vi "Manage_Database.vi"(8 "error in":errorcluster, 10 "To_Do":T1, 11 "All_Communication IN":T2 {"ConfigurationDatabase"."InactivityTime" format="%.0f seconds"; "ConfigurationDatabase"."TravelTime" format="%.0f seconds"; "ConfigurationDatabase"."DoorClose" format="%.0f seconds"; "ConfigurationDatabase"."DoorOpen" format="%.0f seconds"}) -> (0 "error out":errorcluster, 3 "All_Communication OUT":T2 {"ConfigurationDatabase"."InactivityTime" format="%.0f seconds"; "ConfigurationDatabase"."TravelTime" format="%.0f seconds"; "ConfigurationDatabase"."DoorClose" format="%.0f seconds"; "ConfigurationDatabase"."DoorOpen" format="%.0f seconds"})   [LabVIEW 2020]
doc: "Read XML Database, if there is not file load default conf"
uses:
  controls/All_Communication_Data.ctl
  controls/Configuration_Database.ctl
  Message Queue/All Message Queues.ctl
  Message Queue/Message Cluster.ctl
  controls/Event_User.ctl
  Controls/DB_To_do.ctl
  <vilib>/Utility/xml.llb/Write to XML File(string).vi
  <vilib>/Utility/xml.llb/Read From XML File(string).vi
  Message Queue/Message Queue.lvlib
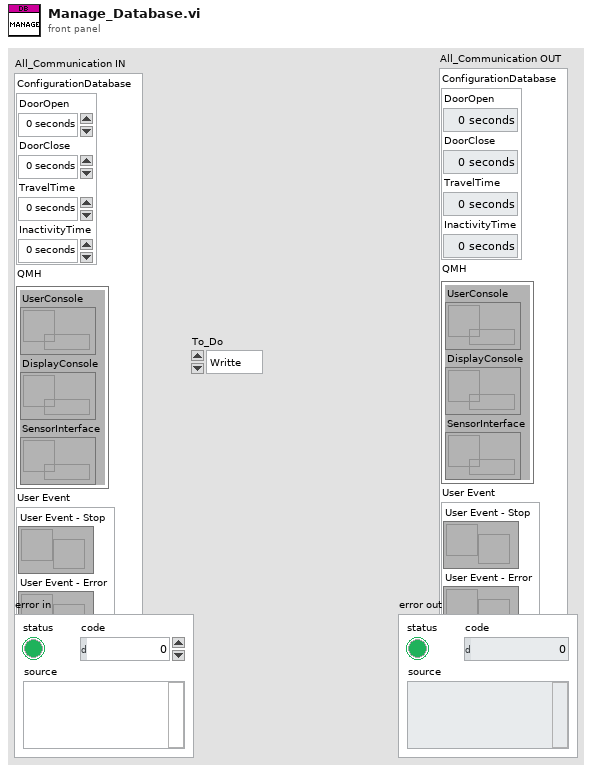
[diagram p1: front panel]
types:
  T1 = typedef "DB_To_do.ctl" = enum16{"Writte", "Read"}
  T2 = typedef "All_Communication_Data.ctl" = cluster{"ConfigurationDatabase":T3, "QMH":T4, "User Event":T5}
  T3 = typedef "Configuration_Database.ctl" = cluster{"DoorOpen":u8, "DoorClose":u8, "TravelTime":u8, "InactivityTime":u8}
  T4 = typedef "Message Queue.lvlib/All Message Queues.ctl" = cluster{"UserConsole":refnum<queue>, "DisplayConsole":refnum<queue>, "SensorInterface":refnum<queue>}
  T5 = typedef "Event_User.ctl" = cluster{"User Event - Stop":refnum<user-event>, "User Event - Error":refnum<user-event>}
  T6 = enum16{"open", "replace", "create", "open or create", "replace or create", "replace or create with confirmation"}
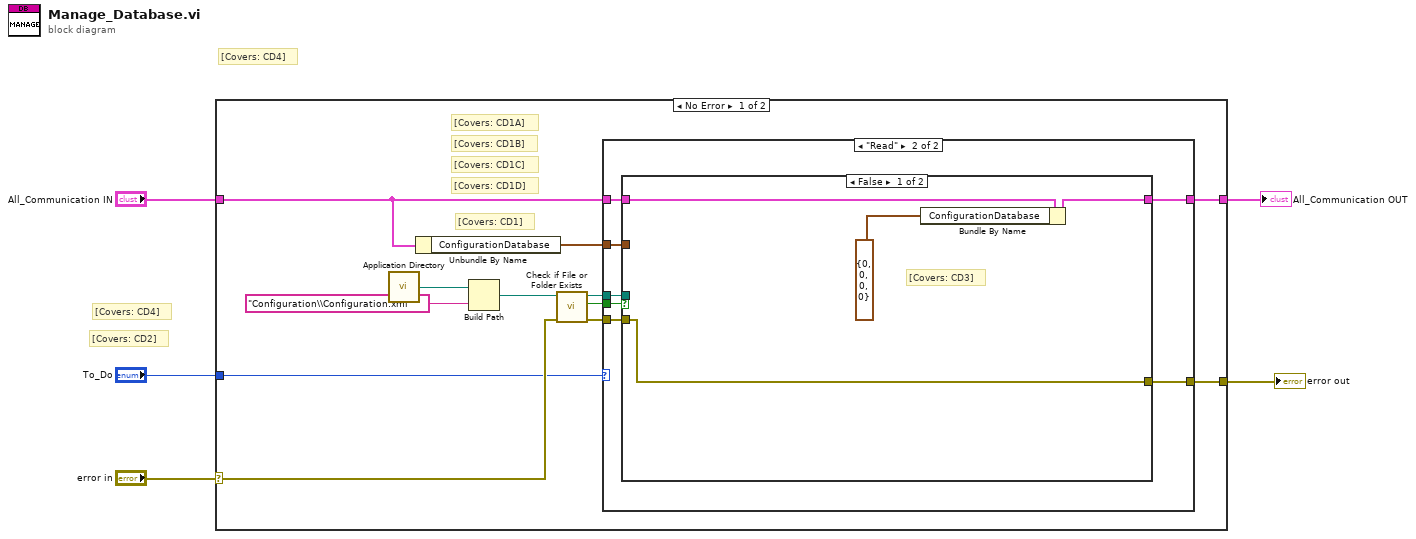
[diagram p0: block diagram]
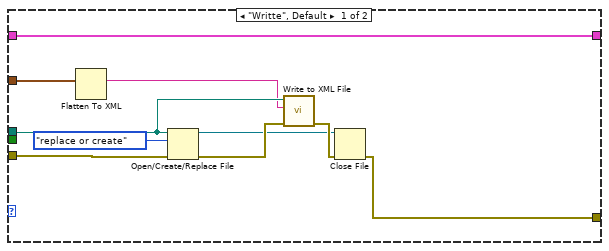
[diagram p2: hidden frame]
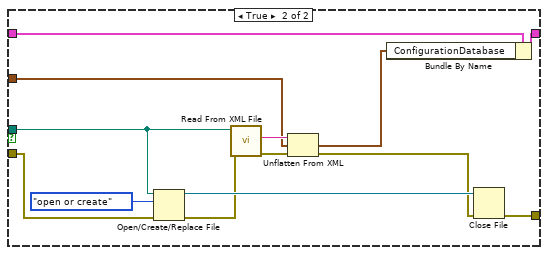
[diagram p3: hidden frame]
diagram:
  # "[Covers: CD4]"
  # "[Covers: CD4]"
  # "[Covers: CD2]"
  n1 = case shown="No Error" "error in" {
    selector: "error in" -> [w14 w52]
    tunnel: "All_Communication IN" -> [w6 w53]
    tunnel: [w17 w52] -> w3
    tunnel: [w9 w53] -> w2
    tunnel: "To_Do" -> [w8 _]
    frame No Error {
      # "[Covers: CD1D]"
      # "[Covers: CD1C]"
      # "[Covers: CD1B]"
      # "[Covers: CD1A]"
      # "[Covers: CD1]"
      n2 = call <vilib>:"Application Directory.vi"() -> ("Application Directory"=w16:path)
      n3 = Unbundle By Name(w6) -> ("ConfigurationDatabase"=w7:T3)
      n4 = Build Path(base path=w16, name or relative path="Configuration\\Configuration.xml") -> (appended path=w13:path)
      n5 = call <vilib>:"Check if File or Folder Exists.vi"("error in (no error)"=w14, "path"=w13) -> ("error out"=w12:errorcluster, "file or folder exists?"=w11:bool, "dup path"=w10:path)  [unwired: 7 in]
      n6 = case shown="\"Read\"" w8 {
        tunnel: [w18 w34] -> w17
        tunnel: w12 -> [w25 w33]
        tunnel: w11 -> [_ w32]
        tunnel: w10 -> [w20 w31]
        tunnel: w6 -> [w27 w30]
        tunnel: [w27 w29] -> w9
        tunnel: w7 -> [w24 w28]
        frame "Writte", Default {
          n7 = Flatten To XML(6:w24) -> (2:w19:string)
          n8 = Open/Create/Replace File(file path (use dialog)=w20, error in=w25, operation (0:open)=T6."replace or create") -> (refnum out=w21:refnum<file>, error out=w23:errorcluster)  [unwired: 3 in, 1 out]
          n9 = call-poly <vilib>:"Write to XML File.vi"("error in (no error)"=w23, "XML Input"=w19, "XML File Path"=w20) -> ("error out"=w22:errorcluster)  [unwired: 6 in, 2 out]
          n10 = Close File(refnum=w21, error in=w22) -> (error out=w18:errorcluster)  [unwired: 1 out]
        }
        frame "Read" {
          n11 = case shown="False" w32 {
            tunnel: [w38 w51] -> w34
            tunnel: w33 -> [w38 w49]
            tunnel: w31 -> [_ w45]
            tunnel: w30 -> [w37 w47]
            tunnel: [w36 w41] -> w29
            tunnel: w28 -> [_ w39]
            frame False {
              # "[Covers: CD3]"
              n12 = Bundle By Name(cluster=w37, "ConfigurationDatabase"=T3 {"DoorOpen"=0, "DoorClose"=0, "TravelTime"=0, "InactivityTime"=0}) -> (w36:T2)
            }
            frame True {
              n13 = Open/Create/Replace File(file path (use dialog)=w45, error in=w49, operation (0:open)=T6."open or create") -> (refnum out=w48:refnum<file>, error out=w46:errorcluster)  [unwired: 3 in, 1 out]
              n14 = call-poly <vilib>:"Read From XML File.vi"("error in (no error)"=w46, "XML File Path"=w45) -> ("error out"=w43:errorcluster, "XML Elements"=w44:string)  [unwired: 7 in, 1 out]
              n15 = Unflatten From XML(xml string=w44, type=w39, error in (no error)=w43) -> (value=w40:T3, error out=w42:errorcluster)
              n16 = Bundle By Name(cluster=w47, "ConfigurationDatabase"=w40) -> (w41:T2)
              n17 = Close File(refnum=w48, error in=w42) -> (error out=w51:errorcluster)  [unwired: 1 out]
            }
          }
        }
      }
    }
    frame Error {
    }
  }
  "All_Communication OUT" <- w2
  "error out" <- w3
